vi "FTW-TransferClient-dotNET-CreateURI.vi"(0 "URI":string, 5 "Relative URI":string, 11 "error in":errorcluster) -> (4 "URI ref":refnum<k24>, 6 "Host":string, 8 "Scheme":string, 10 "AbsoluteURI":string, 14 "Segments":string[](array[string]), 15 "error out":errorcluster)   [LabVIEW 2013, in "FTW-TransferClient-dotNET.lvclass"]
uses:
  FTW-TransferClient-dotNET.lvclass
panel:
  # "Inputs"
  # "Outputs"
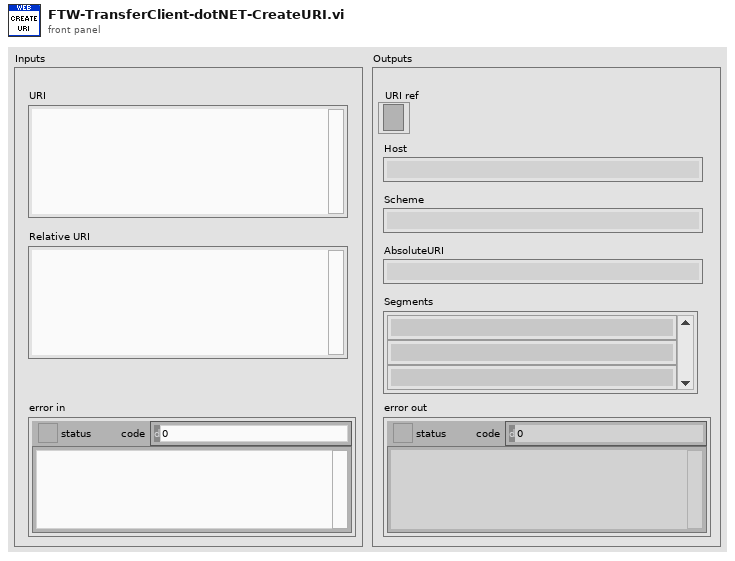
[diagram p1: front panel]
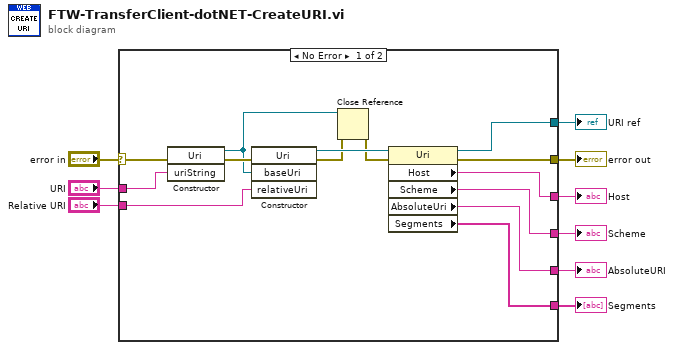
[diagram p0: block diagram]
diagram:
  n1 = case shown="No Error" "error in" {
    selector: "error in" -> [w14 w24]
    tunnel: [w21 w24] -> w9
    tunnel: [w22 _] -> w8
    tunnel: "URI" -> [w16 _]
    tunnel: [w20 _] -> w5
    tunnel: [w19 _] -> w4
    tunnel: [w18 _] -> w3
    tunnel: [w17 _] -> w2
    tunnel: "Relative URI" -> [w15 _]
    frame No Error {
      n2 = constructor class="Uri"(error in=w14, "uriString"=w16) -> (reference out=w12:refnum<k24>, error out=w13:errorcluster)  [unwired: 2 in, 2 out]
      n3 = constructor class="Uri"(error in=w13, "baseUri"=w12, "relativeUri"=w15) -> (reference out=w23:refnum<k24>, error out=w11:errorcluster)  [unwired: 2 in, 3 out]
      n4 = Close Reference(reference=w12, error in (no error)=w11) -> (error out=w10:errorcluster)
      n5 = property class="Uri"(reference=w23, error in=w10) -> (reference out=w22:refnum<k24>, error out=w21:errorcluster, "Host"=w19:string, "Scheme"=w20:string, "AbsoluteUri"=w18:string, "Segments"=w17:string[])
    }
    frame Error {
    }
  }
  "error out" <- w9
  "URI ref" <- w8
  "Scheme" <- w5
  "Host" <- w4
  "AbsoluteURI" <- w3
  "Segments" <- w2
